vi "Write data.vi"(8 "error in (no error)":errorcluster, 10 "data":cluster{"Socket":i32, "Info":string}, 11 "Exit in":refnum<class "Exit.lvclass">) -> (0 "error out":errorcluster, 3 "Exit out":refnum<class "Exit.lvclass">)   [LabVIEW 2019, in "SignalProcessing.lvlib" / "Exit.lvclass"]
uses:
  Exit.lvclass
  Exit.lvclass/Exit.ctl
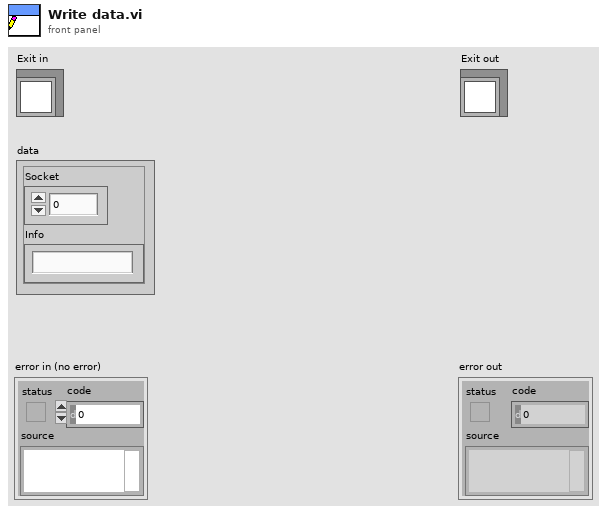
[diagram p1: front panel]
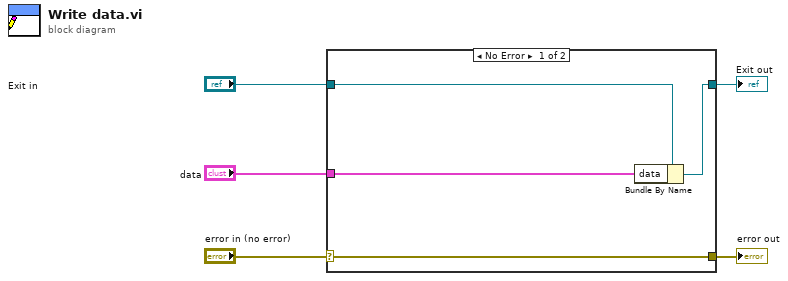
[diagram p0: block diagram]
diagram:
  n1 = case shown="No Error" "error in (no error)" {
    selector: "error in (no error)" -> [w9 w10]
    tunnel: [w9 w10] -> w4
    tunnel: [w7 w11] -> w2
    tunnel: "Exit in" -> [w8 w11]
    tunnel: "data" -> [w6 _]
    frame No Error {
      n2 = Bundle By Name(cluster=w8, "data"=w6) -> (w7:refnum<class "Exit.lvclass">)
    }
    frame Error {
    }
  }
  "error out" <- w4
  "Exit out" <- w2
